vi "Remote - ExecuteEvent.vi"(0 "LVx Command in":refnum<class "LVx.lvclass">, 1 "application reference":refnum<vi>, 5 "Session ID":string, 11 "error in (no error)":errorcluster, 12 "Retain Session (F)":bool) -> (4 "LVx Command out":refnum<class "LVx.lvclass">, 15 "error out":errorcluster)   [LabVIEW 2011, in "LVx.lvlib" / "LVx.lvclass"]
uses:
  LVx.lvclass
  LVx.lvlib
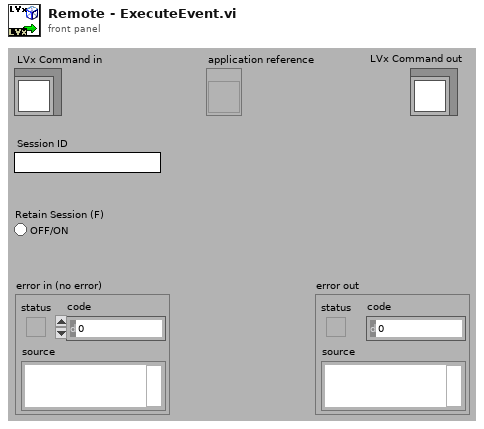
[diagram p1: front panel]
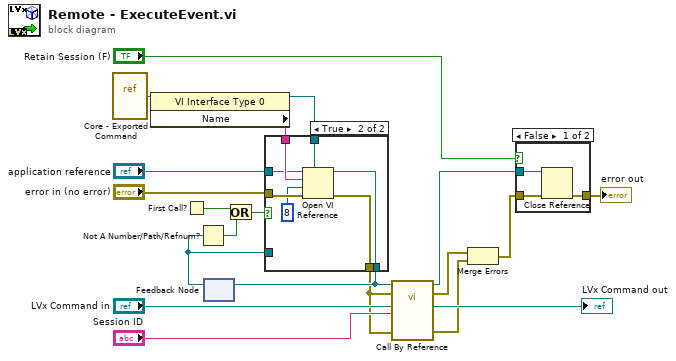
[diagram p0: block diagram]
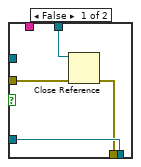
[diagram p3: hidden frame]
diagram:
  n1 = vi-ref "Core - Exported Command.vi"() -> (w15:refnum<vi>)
  n2 = property class="VI Interface Type 0"(reference=w15) -> (reference out=w17:refnum<vi>, "Name"=w1:string)  [unwired: 1 in, 1 out]
  n3 = First Call?() -> (First Call?: T/F=w4:bool)
  n4 = feedback #1() -> (w2:refnum<vi>)  [unwired: 1 out]
  n5 = Not A Number/Path/Refnum?(number/path/refnum=w2) -> (NaN/Path/Refnum?=w3:bool)
  n6 = Or(x=w4, y=w3) -> (x .or. y?=w5:bool)
  n7 = case shown="True" w5 {
    tunnel: [w24 w31] -> w11
    tunnel: w1 -> [_ w30]
    tunnel: w17 -> [w23 w29]
    tunnel: "application reference" -> [_ w28]
    tunnel: "error in (no error)" -> [w22 w27]
    tunnel: [w21 w26] -> w7
    tunnel: w2 -> [w24 _]
    frame False {
      n8 = Close Reference(reference=w23, error in (no error)=w22) -> (error out=w21:errorcluster)
    }
    frame True {
      n9 = Open VI Reference(type specifier VI Refnum (for type only)=w29, application reference (local)=w28, vi path=w30, options=8, error in (no error)=w27) -> (vi reference=w31:refnum<vi>, error out=w26:errorcluster)  [unwired: 1 out]
    }
  }
  n10 = feedback-in #1(w11) -> ()
  n11 = call-by-ref "?"(reference=w11, error in=w7, "LVx Command in"="LVx Command in", "Session ID"="Session ID", 11:"error in (no error)"=w7) -> (reference out=w18:refnum<vi>, error out=w12:errorcluster, "LVx Command out"=→"LVx Command out":refnum<class "LVx.lvclass">, 15:"error out"=w6:errorcluster)  [unwired: 10 in, 1 out]
  n12 = Merge Errors(w12, w6) -> (w19:errorcluster)
  n13 = case shown="False" "Retain Session (F)" {
    tunnel: w19 -> [w34 w35]
    tunnel: w18 -> [w33 _]
    tunnel: [w32 w35] -> w14
    frame False {
      n14 = Close Reference(reference=w33, error in (no error)=w34) -> (error out=w32:errorcluster)
    }
    frame True {
    }
  }
  "error out" <- w14
